vi "Power Output Measurements Key Array.vi"(4 "Conversion":enum16{"Cluster - HTML", "HTML - Cluster"}(ring), 6 "Measurements Key Array In":T5, 7 "Measurements Cluster In":T1 {"Frequency Step Size" items=["0.2", "0.4", "1.0", "2.0", "4.0"]; "Direction" items=["Reverse", "Forward", "Auxiliary"]}) -> (1 "Measurements Cluster Out":T1 {"Frequency Step Size" items=["0.2", "0.4", "1.0", "2.0", "4.0"]; "Direction" items=["Reverse", "Forward", "Auxiliary"]}, 2 "Measurements HTML Out":string)   [LabVIEW 2011]
uses:
  Addons/internet/utils/keyedarr.llb/Keyed Array.ctl
  TypeDefs/Power Output Measurement Parameters.ctl
  SI.LIB/PIM.LIB/HW IO/DUTport.ctl
  SI.LIB/PIM.LIB/HW IO/MeasMode.ctl
  SI.LIB/PIM.LIB/HW IO/PIM Sweep Step Size.ctl
  Addons/internet/utils/strutil.llb/Case Matching.ctl
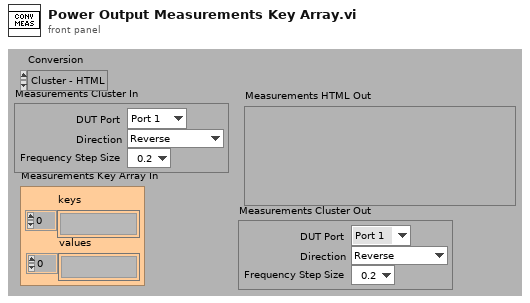
[diagram p1: front panel]
types:
  T1 = typedef "Power Output Measurement Parameters.ctl" = cluster{"DUT Port":T2, "Direction":T3, "Frequency Step Size":T4}
  T2 = typedef "DUTport.ctl" = enum16{"Port 1", "Port 2"}
  T3 = typedef "MeasMode.ctl" = u16
  T4 = typedef "PIM Sweep Step Size.ctl" = u16
  T5 = typedef "Keyed Array.ctl" = cluster{"keys":string[], "values":string[]}
  T6 = typedef "Case Matching.ctl" = enum16{"a != A", "a == A", "system"}
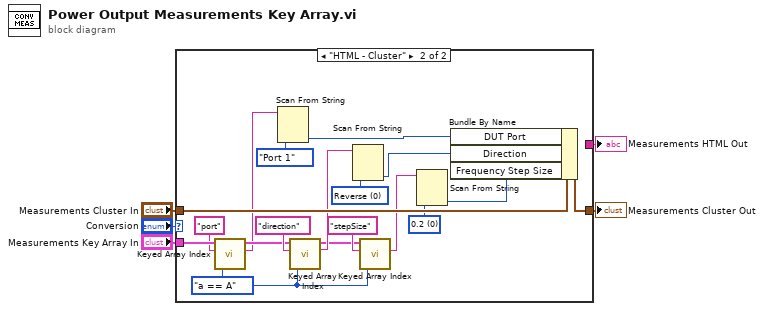
[diagram p0: block diagram]
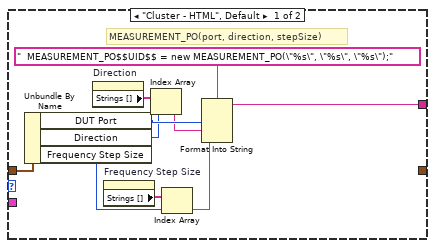
[diagram p2: hidden frame]
diagram:
  n1 = case shown="\"HTML - Cluster\"" "Conversion" {
    tunnel: "Measurements Key Array In" -> [_ w33]
    tunnel: "Measurements Cluster In" -> [w15 w31]
    tunnel: [_ w30] -> w3
    tunnel: [w12 _] -> w1
    frame "Cluster - HTML", Default {
      # "MEASUREMENT_PO(port, direction, stepSize)"
      n2 = Unbundle By Name(w15) -> ("DUT Port"=w13:T2, "Direction"=w11:T3, "Frequency Step Size"=w7:T4)
      n3 = property on="Direction" class="Ring (strict)"() -> ("Strings []"=w10:string[])  [unwired: 2 in, 2 out]
      n4 = property on="Frequency Step Size" class="Ring (strict)"() -> ("Strings []"=w8:string[])  [unwired: 2 in, 2 out]
      n5 = Index Array(array=w10, index=w11) -> (element=w9:string)
      n6 = Index Array(array=w8, index=w7) -> (element=w6:string)
      n7 = Format Into String(format string="  MEASUREMENT_PO$$UID$$ = new MEASUREMENT_PO(\"%s\", \"%s\", \"%s\");", w13, w9, w6) -> (resulting string=w12:string)  [unwired: 2 in, 1 out]
    }
    frame "HTML - Cluster" {
      w18 = T4 0 items=["0.2", "0.4", "1.0", "2.0", "4.0"] ("Frequency Step Size")
      w19 = T3 0 items=["Reverse", "Forward", "Auxiliary"] ("Direction")
      w20 = Case_Matching."a == A" ("case matching (sensitive)")
      n8 = call "Keyed Array Index.vi"("case matching (sensitive)"=w20, "key"="port", "array in"=w33) -> ("value"=w25:string, "duplicate array"=w28:T5)  [unwired: 1 in, 2 out]
      n9 = Scan From String(input string=w25, default 1=DUTport."Port 1" ("Measure.DUT PORT")) -> (output 1=w24:T2)  [unwired: 3 in, 3 out]
      n10 = call "Keyed Array Index.vi"("case matching (sensitive)"=w20, "key"="direction", "array in"=w28) -> ("value"=w27:string, "duplicate array"=w21:T5)  [unwired: 1 in, 2 out]
      n11 = Scan From String(input string=w27, default 1=w19) -> (output 1=w23:T3)  [unwired: 3 in, 3 out]
      n12 = call "Keyed Array Index.vi"("case matching (sensitive)"=w20, "key"="stepSize", "array in"=w21) -> ("value"=w17:string)  [unwired: 1 in, 3 out]
      n13 = Scan From String(input string=w17, default 1=w18) -> (output 1=w16:T4)  [unwired: 3 in, 3 out]
      n14 = Bundle By Name(cluster=w31, "DUT Port"=w24, "Direction"=w23, "Frequency Step Size"=w16) -> (w30:T1)
    }
  }
  "Measurements HTML Out" <- w1
  "Measurements Cluster Out" <- w3
